vi "Handle.vi"(11 "Base Event in":refnum<class "Base Event.lvclass">) -> (2 "Destroy?":bool, 3 "Base Event out":refnum<class "Base Event.lvclass">)   [LabVIEW 2021, in "jettl.lvlib" / "Base Event.lvlib" / "Base Event.lvclass"]
uses:
  Base Event.lvclass
  C:/git/jettl/jettl/jettl/Event/Event.lvclass
  State/Error State/Error State.lvclass
  C:/git/jettl/jettl/jettl/Base Event/State/State/State.lvclass
  Base Event.lvclass/Base Event.ctl
  State/Nominal State/Nominal State.lvclass
  C:/git/jettl/jettl/jettl/Base Event/State/Error State/Error State.lvclass
  C:/git/jettl/jettl/jettl/Base Event/State/Nominal State/Nominal State.lvclass
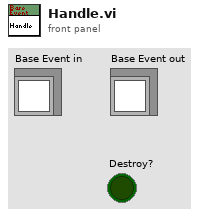
[diagram p1: front panel]
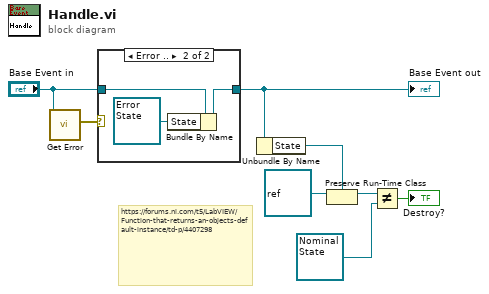
[diagram p0: block diagram]
diagram:
  # "https://forums.ni.com/t5/LabVIEW/Function-that-returns-an-objects-default-instance/td-p/4407298"
  n1 = call-dynamic "Get Error.vi"("Base Event in"="Base Event in") -> ("Error"=w8:errorcluster)  [unwired: 10 in]
  n2 = case shown="Error .." w8 {
    tunnel: [w9 w11] -> w6
    tunnel: "Base Event in" -> [w9 w12]
    frame No Error {
    }
    frame Error {
      n3 = Bundle By Name(cluster=w12, "State"=refnum<class "Error State.lvclass"> refnum ("jettl.lvlib:Error Event State.lvclass")) -> (w11:refnum<class "Base Event.lvclass">)
    }
  }
  "Base Event out" <- w6
  n4 = Unbundle By Name(w6) -> ("State"=w3:refnum<class "State.lvclass">)
  n5 = Preserve Run-Time Class(object in=refnum<class> refnum ("LabVIEW Object"), 2:w3) -> (object out=w4:refnum<class "State.lvclass">)  [unwired: 1 in, 1 out]
  n6 = Not Equal?(x=w4, y=refnum<class "Nominal State.lvclass"> refnum ("jettl.lvlib:Base Event.lvlib:State.lvlib:Nominal State.lvclass")) -> (x != y?=→"Destroy?":bool)
